vi "状态告警区.vi"(11 "数组":u16[](array[numeric]) format="%04xH") -> (2 "状态告警区 2":T1 {"工作状态" items=["空闲"=0, "水样测试"=1, "标样核查"=2, "零点核查"=3, "跨度核查"=4, "空白测试"=5, "平行样测试"=6, "加标回收"=7, "空白校准"=8, "标样校准"=9, "初始化（清洗）"=10, "单步调试"=254, "简易步骤"=255]; "告警代码" items=["无告警", "缺试剂告警", "缺水样告警", "缺蒸馏水告警", "缺标液告警", "仪表漏液告警", "标定异常告警", "超量程告警", "加热异常", "低试剂预警", "超上限告警", "超下限告警", "仪表内部其他异常", "滴定异常告警", "电极异常告警", "量程切换告警", "参数设置告警", "PH电极电位异常", "电导率电极异常", "浊度光度异常", "溶解氧电极异常", "溶解氧光强异常", "温度异常告警", "PH异常告警", "溶解氧异常告警", "电导率异常告警", "浊度异常告警", "叶绿素异常告警", "藻密度异常告警", "蓝绿藻异常告警", "ORP异常告警", "氨氮异常告警", "清洁刷异常告警", "SD卡异常告警", "蓝牙异常告警", "Wifi异常告警", "流程异常告警"]; "故障代码" items=["无故障", "电机故障", "温度故障", "通讯故障", "滴定故障"]}, 3 "状态告警区":T2 {"工作状态" items=["空闲"=0, "水样测试"=1, "标样核查"=2, "零点核查"=3, "跨度核查"=4, "空白测试"=5, "平行样测试"=6, "加标回收"=7, "空白校准"=8, "标样校准"=9, "初始化（清洗）"=10, "单步调试"=254, "简易步骤"=255]; "告警代码" items=["无告警", "缺试剂告警", "缺水样告警", "缺蒸馏水告警", "缺标液告警", "仪表漏液告警", "标定异常告警", "超量程告警", "加热异常", "低试剂预警", "超上限告警", "超下限告警", "仪表内部其他异常", "滴定异常告警", "电极异常告警", "量程切换告警", "参数设置告警", "PH电极电位异常", "电导率电极异常", "浊度光度异常", "溶解氧电极异常", "溶解氧光强异常", "温度异常告警", "PH异常告警", "溶解氧异常告警", "电导率异常告警", "浊度异常告警", "叶绿素异常告警", "藻密度异常告警", "蓝绿藻异常告警", "ORP异常告警", "氨氮异常告警", "清洁刷异常告警", "SD卡异常告警", "蓝牙异常告警", "Wifi异常告警", "流程异常告警"]; "故障代码" items=["无故障", "电机故障", "温度故障", "通讯故障", "滴定故障"]})   [LabVIEW 2022 SP3, in "斯坦道总氮.lvlib"]
panel:
  # "共占用29 WORD"
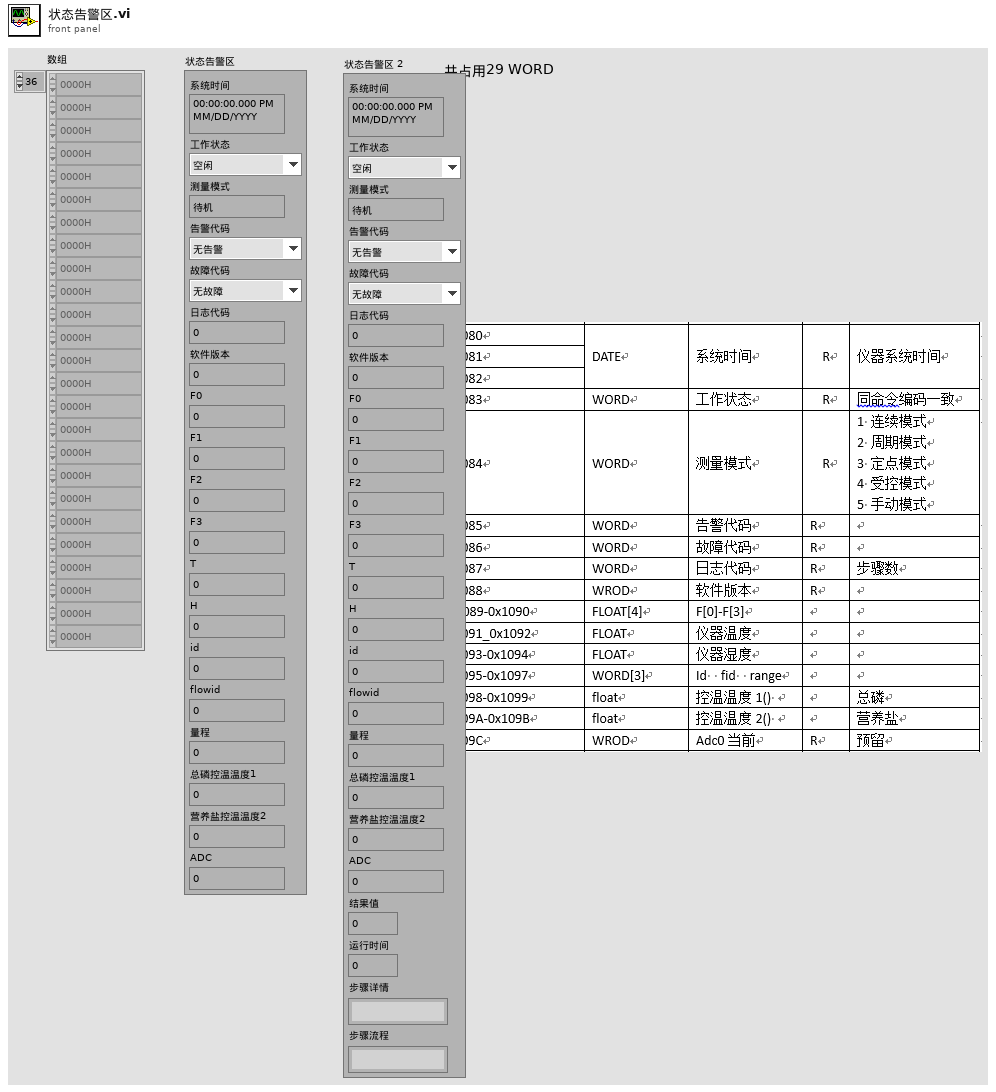
[diagram p1: front panel]
types:
  T1 = cluster{"系统时间":timestamp, "工作状态":u16, "测量模式":enum16{"待机", "连续模式", "周期模式", "定点模式", "受控模式", "手动模式"}, "告警代码":u16, "故障代码":u16, "日志代码":u16, "软件版本":u16, "F0":sgl, "F1":sgl, "F2":sgl, "F3":sgl, "T":sgl, "H":sgl, "id":u16, "flowid":u16, "量程":u16, "总磷控温温度1":sgl, "营养盐控温温度2":sgl, "ADC":sgl, "结果值":sgl, "运行时间":u16, "步骤详情":string, "步骤流程":string}
  T2 = cluster{"系统时间":timestamp, "工作状态":u16, "测量模式":enum16{"待机", "连续模式", "周期模式", "定点模式", "受控模式", "手动模式"}, "告警代码":u16, "故障代码":u16, "日志代码":u16, "软件版本":u16, "F0":sgl, "F1":sgl, "F2":sgl, "F3":sgl, "T":sgl, "H":sgl, "id":u16, "flowid":u16, "量程":u16, "总磷控温温度1":sgl, "营养盐控温温度2":sgl, "ADC":sgl}
  T3 = enum16{"待机", "连续模式", "周期模式", "定点模式", "受控模式", "手动模式"}
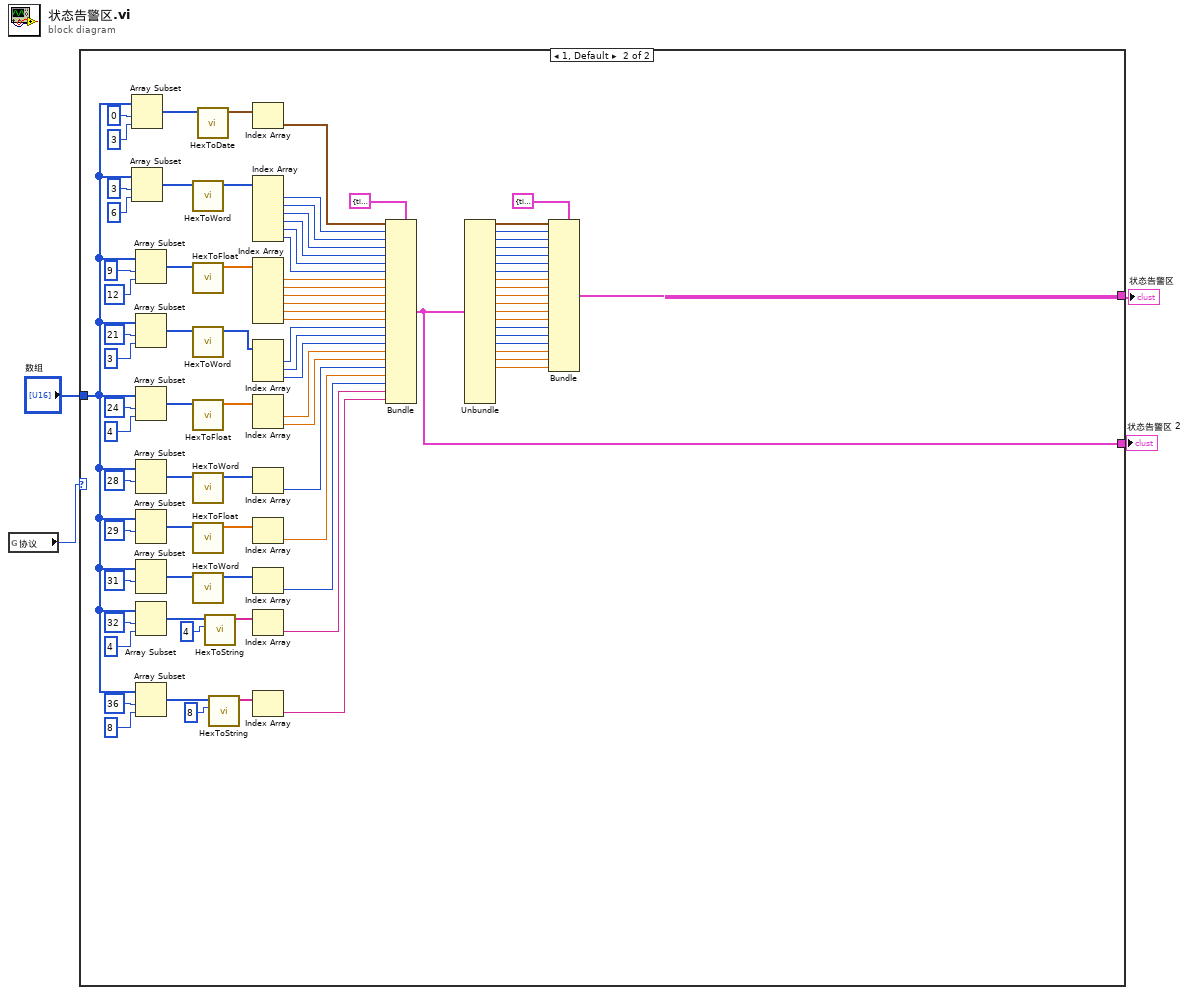
[diagram p0: block diagram]
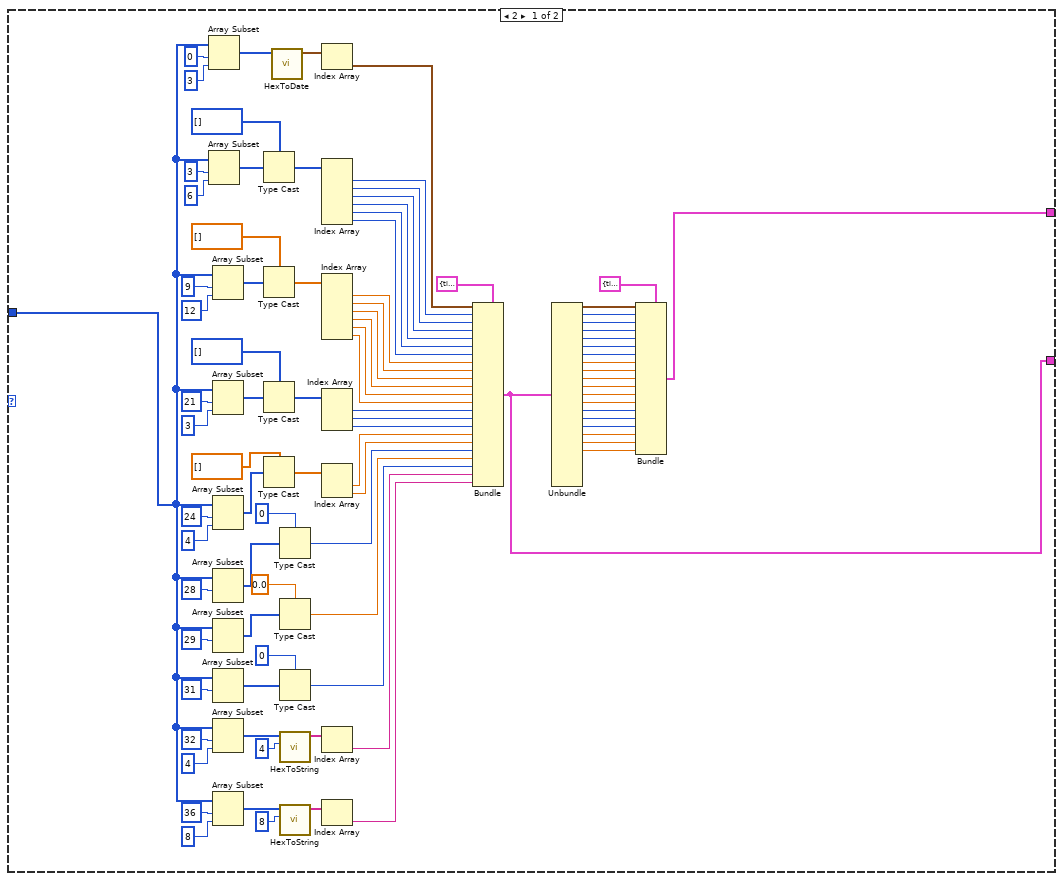
[diagram p2: hidden frame]
diagram:
  n1 = global read "总磷总氮断电保存全局变量.vi" "协议"() -> (w1:u16)
  n2 = case shown="1, Default" w1 {
    tunnel: [w5 w137] -> w4
    tunnel: [w6 w116] -> w3
    tunnel: "数组" -> [w7 w96]
    frame 2 {
      n3 = Array Subset(array=w7, index=0 ("索引"), length=3 ("长度")) -> (w92:u16[])
      n4 = Array Subset(array=w7, index=3 ("索引"), length=6 ("长度")) -> (w28:u16[])
      n5 = Array Subset(array=w7, index=9 ("索引"), length=12 ("长度")) -> (w24:u16[])
      n6 = Array Subset(array=w7, index=21 ("索引"), length=3 ("索引")) -> (w21:u16[])
      n7 = Array Subset(array=w7, index=24 ("索引"), length=4 ("索引")) -> (w15:u16[])
      n8 = Array Subset(array=w7, index=28 ("索引")) -> (w18:u16[])  [unwired: 1 in]
      n9 = Array Subset(array=w7, index=29 ("索引")) -> (w13:u16[])  [unwired: 1 in]
      n10 = Array Subset(array=w7, index=31 ("索引")) -> (w9:u16[])  [unwired: 1 in]
      n11 = Array Subset(array=w7, index=32 ("索引"), length=4 ("长度")) -> (w39:u16[])
      n12 = Array Subset(array=w7, index=36 ("索引"), length=8 ("长度")) -> (w31:u16[])
      n13 = Type Cast(type=u16[] [], x=w28) -> (*(type *) &x=w26:u16[])
      n14 = Type Cast(type=sgl[] [], x=w24) -> (*(type *) &x=w23:sgl[])
      n15 = Type Cast(type=u16[] [], x=w21) -> (*(type *) &x=w20:u16[])
      n16 = Type Cast(type=sgl[] [], x=w15) -> (*(type *) &x=w14:sgl[])
      n17 = call "HexToDate.vi"("数组"=w92) -> ("DATE"=w89:timestamp[])  [unwired: 10 in]
      n18 = Type Cast(type=u16 0, x=w18) -> (*(type *) &x=w17:u16)
      n19 = Type Cast(type=sgl 0.0, x=w13) -> (*(type *) &x=w11:sgl)
      n20 = Type Cast(type=u16 0, x=w9) -> (*(type *) &x=w8:u16)
      n21 = call "HexToString.vi"("字符个数"=4, "数组"=w39) -> ("STRING"=w37:string[])  [unwired: 9 in]
      n22 = call "HexToString.vi"("字符个数"=8, "数组"=w31) -> ("STRING"=w33:string[])  [unwired: 9 in]
      n23 = Index Array(array=w89) -> (element=w88:timestamp)  [unwired: 1 in]
      n24 = Index Array(array=w26) -> (element #1=w87:u16, element #2=w86:u16, element #3=w85:u16, element #4=w84:u16, element #5=w83:u16, element #6=w82:u16)  [unwired: 6 in]
      n25 = Index Array(array=w23) -> (element #1=w79:sgl, element #2=w78:sgl, element #3=w77:sgl, element #4=w76:sgl, element #5=w75:sgl, element #6=w74:sgl)  [unwired: 6 in]
      n26 = Index Array(array=w20) -> (element #1=w71:u16, element #2=w70:u16, element #3=w69:u16)  [unwired: 3 in]
      n27 = Index Array(array=w14) -> (element #1=w66:sgl, element #2=w65:sgl)  [unwired: 2 in]
      n28 = Index Array(array=w37) -> (element=w36:string)  [unwired: 1 in]
      n29 = Index Array(array=w33) -> (element=w29:string)  [unwired: 1 in]
      n30 = Bundle(cluster=T1 {"系统时间"=timestamp(0 s since 1904-01-01), "工作状态"=0, "测量模式"=enum."待机", "告警代码"=0, "故障代码"=0, "日志代码"=0, "软件版本"=0, "F0"=0.0, "F1"=0.0, "F2"=0.0, "F3"=0.0, "T"=0.0, "H"=0.0, "id"=0, "flowid"=0, "量程"=0, "总磷控温温度1"=0.0, "营养盐控温温度2"=0.0, "ADC"=0.0, "结果值"=0.0, "运行时间"=0, "步骤详情"="", "步骤流程"=""} ("状态告警区 2"), "系统时间"=w88, "工作状态"=w87, "测量模式"=w86, "告警代码"=w85, "故障代码"=w84, "日志代码"=w83, "软件版本"=w82, "F0"=w79, "F1"=w78, "F2"=w77, "F3"=w76, "T"=w75, "H"=w74, "id"=w71, "flowid"=w70, "量程"=w69, "总磷控温温度1"=w66, "营养盐控温温度2"=w65, "ADC"=w17, "结果值"=w11, "运行时间"=w8, "步骤详情"=w36, "步骤流程"=w29) -> (w5:T1)
      n31 = Unbundle(w5) -> ("系统时间"=w61:timestamp, "工作状态"=w60:u16, "测量模式"=w59:T3, "告警代码"=w58:u16, "故障代码"=w57:u16, "日志代码"=w56:u16, "软件版本"=w55:u16, "F0"=w54:sgl, "F1"=w53:sgl, "F2"=w52:sgl, "F3"=w51:sgl, "T"=w50:sgl, "H"=w49:sgl, "id"=w48:u16, "flowid"=w47:u16, "量程"=w46:u16, "总磷控温温度1"=w45:sgl, "营养盐控温温度2"=w44:sgl, "ADC"=w43:sgl)  [unwired: 4 out]
      n32 = Bundle(cluster=T2 {"系统时间"=timestamp(0 s since 1904-01-01), "工作状态"=0, "测量模式"=enum."待机", "告警代码"=0, "故障代码"=0, "日志代码"=0, "软件版本"=0, "F0"=0.0, "F1"=0.0, "F2"=0.0, "F3"=0.0, "T"=0.0, "H"=0.0, "id"=0, "flowid"=0, "量程"=0, "总磷控温温度1"=0.0, "营养盐控温温度2"=0.0, "ADC"=0.0} ("状态告警区"), "系统时间"=w61, "工作状态"=w60, "测量模式"=w59, "告警代码"=w58, "故障代码"=w57, "日志代码"=w56, "软件版本"=w55, "F0"=w54, "F1"=w53, "F2"=w52, "F3"=w51, "T"=w50, "H"=w49, "id"=w48, "flowid"=w47, "量程"=w46, "总磷控温温度1"=w45, "营养盐控温温度2"=w44, "ADC"=w43) -> (w6:T2)
    }
    frame 1, Default {
      n33 = Array Subset(array=w96, index=0 ("索引"), length=3 ("长度")) -> (w178:u16[])
      n34 = Array Subset(array=w96, index=3 ("索引"), length=6 ("长度")) -> (w173:u16[])
      n35 = Array Subset(array=w96, index=9 ("索引"), length=12 ("长度")) -> (w163:u16[])
      n36 = Array Subset(array=w96, index=21 ("索引"), length=3 ("索引")) -> (w153:u16[])
      n37 = Array Subset(array=w96, index=24 ("索引"), length=4 ("索引")) -> (w146:u16[])
      n38 = Array Subset(array=w96, index=28 ("索引")) -> (w141:u16[])  [unwired: 1 in]
      n39 = Array Subset(array=w96, index=29 ("索引")) -> (w114:u16[])  [unwired: 1 in]
      n40 = Array Subset(array=w96, index=31 ("索引")) -> (w110:u16[])  [unwired: 1 in]
      n41 = Array Subset(array=w96, index=32 ("索引"), length=4 ("长度")) -> (w106:u16[])
      n42 = Array Subset(array=w96, index=36 ("索引"), length=8 ("长度")) -> (w98:u16[])
      n43 = call "HexToWord.vi"("数组"=w173) -> ("WORD"=w172:u16[])  [unwired: 10 in]
      n44 = call "HexToFloat.vi"("数组"=w163) -> ("FLOAT"=w162:sgl[])  [unwired: 10 in]
      n45 = call "HexToWord.vi"("数组"=w153) -> ("WORD"=w152:u16[])  [unwired: 10 in]
      n46 = call "HexToFloat.vi"("数组"=w146) -> ("FLOAT"=w145:sgl[])  [unwired: 10 in]
      n47 = call "HexToWord.vi"("数组"=w141) -> ("WORD"=w142:u16[])  [unwired: 10 in]
      n48 = call "HexToFloat.vi"("数组"=w114) -> ("FLOAT"=w113:sgl[])  [unwired: 10 in]
      n49 = call "HexToWord.vi"("数组"=w110) -> ("WORD"=w109:u16[])  [unwired: 10 in]
      n50 = call "HexToDate.vi"("数组"=w178) -> ("DATE"=w175:timestamp[])  [unwired: 10 in]
      n51 = call "HexToString.vi"("字符个数"=4, "数组"=w106) -> ("STRING"=w104:string[])  [unwired: 9 in]
      n52 = call "HexToString.vi"("字符个数"=8, "数组"=w98) -> ("STRING"=w100:string[])  [unwired: 9 in]
      n53 = Index Array(array=w175) -> (element=w174:timestamp)  [unwired: 1 in]
      n54 = Index Array(array=w172) -> (element #1=w171:u16, element #2=w170:u16, element #3=w169:u16, element #4=w168:u16, element #5=w167:u16, element #6=w166:u16)  [unwired: 6 in]
      n55 = Index Array(array=w162) -> (element #1=w161:sgl, element #2=w160:sgl, element #3=w159:sgl, element #4=w158:sgl, element #5=w157:sgl, element #6=w156:sgl)  [unwired: 6 in]
      n56 = Index Array(array=w152) -> (element #1=w151:u16, element #2=w150:u16, element #3=w149:u16)  [unwired: 3 in]
      n57 = Index Array(array=w145) -> (element #1=w144:sgl, element #2=w143:sgl)  [unwired: 2 in]
      n58 = Index Array(array=w142) -> (element=w139:u16)  [unwired: 1 in]
      n59 = Index Array(array=w113) -> (element=w112:sgl)  [unwired: 1 in]
      n60 = Index Array(array=w109) -> (element=w108:u16)  [unwired: 1 in]
      n61 = Index Array(array=w104) -> (element=w103:string)  [unwired: 1 in]
      n62 = Index Array(array=w100) -> (element=w95:string)  [unwired: 1 in]
      n63 = Bundle(cluster=T1 {"系统时间"=timestamp(0 s since 1904-01-01), "工作状态"=0, "测量模式"=enum."待机", "告警代码"=0, "故障代码"=0, "日志代码"=0, "软件版本"=0, "F0"=0.0, "F1"=0.0, "F2"=0.0, "F3"=0.0, "T"=0.0, "H"=0.0, "id"=0, "flowid"=0, "量程"=0, "总磷控温温度1"=0.0, "营养盐控温温度2"=0.0, "ADC"=0.0, "结果值"=0.0, "运行时间"=0, "步骤详情"="", "步骤流程"=""} ("状态告警区 2"), "系统时间"=w174, "工作状态"=w171, "测量模式"=w170, "告警代码"=w169, "故障代码"=w168, "日志代码"=w167, "软件版本"=w166, "F0"=w161, "F1"=w160, "F2"=w159, "F3"=w158, "T"=w157, "H"=w156, "id"=w151, "flowid"=w150, "量程"=w149, "总磷控温温度1"=w144, "营养盐控温温度2"=w143, "ADC"=w139, "结果值"=w112, "运行时间"=w108, "步骤详情"=w103, "步骤流程"=w95) -> (w137:T1)
      n64 = Unbundle(w137) -> ("系统时间"=w135:timestamp, "工作状态"=w134:u16, "测量模式"=w133:T3, "告警代码"=w132:u16, "故障代码"=w131:u16, "日志代码"=w130:u16, "软件版本"=w129:u16, "F0"=w128:sgl, "F1"=w127:sgl, "F2"=w126:sgl, "F3"=w125:sgl, "T"=w124:sgl, "H"=w123:sgl, "id"=w122:u16, "flowid"=w121:u16, "量程"=w120:u16, "总磷控温温度1"=w119:sgl, "营养盐控温温度2"=w118:sgl, "ADC"=w117:sgl)  [unwired: 4 out]
      n65 = Bundle(cluster=T2 {"系统时间"=timestamp(0 s since 1904-01-01), "工作状态"=0, "测量模式"=enum."待机", "告警代码"=0, "故障代码"=0, "日志代码"=0, "软件版本"=0, "F0"=0.0, "F1"=0.0, "F2"=0.0, "F3"=0.0, "T"=0.0, "H"=0.0, "id"=0, "flowid"=0, "量程"=0, "总磷控温温度1"=0.0, "营养盐控温温度2"=0.0, "ADC"=0.0} ("状态告警区"), "系统时间"=w135, "工作状态"=w134, "测量模式"=w133, "告警代码"=w132, "故障代码"=w131, "日志代码"=w130, "软件版本"=w129, "F0"=w128, "F1"=w127, "F2"=w126, "F3"=w125, "T"=w124, "H"=w123, "id"=w122, "flowid"=w121, "量程"=w120, "总磷控温温度1"=w119, "营养盐控温温度2"=w118, "ADC"=w117) -> (w116:T2)
    }
  }
  "状态告警区" <- w3
  "状态告警区 2" <- w4
